vi "out_dc_unit.vi"(1 "input":T1) -> (0 "output":T2)   [LabVIEW 2013]
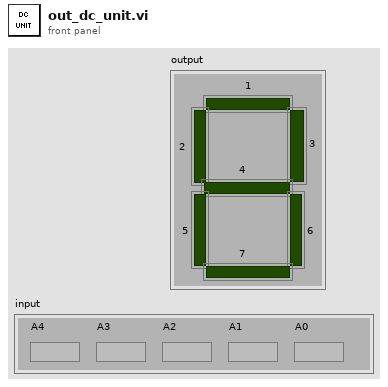
[diagram p1: front panel]
types:
  T1 = cluster{"A4":bool, "A3":bool, "A2":bool, "A1":bool, "A0":bool}
  T2 = cluster{"1":bool, "2":bool, "3":bool, "4":bool, "5":bool, "6":bool, "7":bool}
  T3 = cluster{bool, bool, bool, bool, bool, bool, bool}
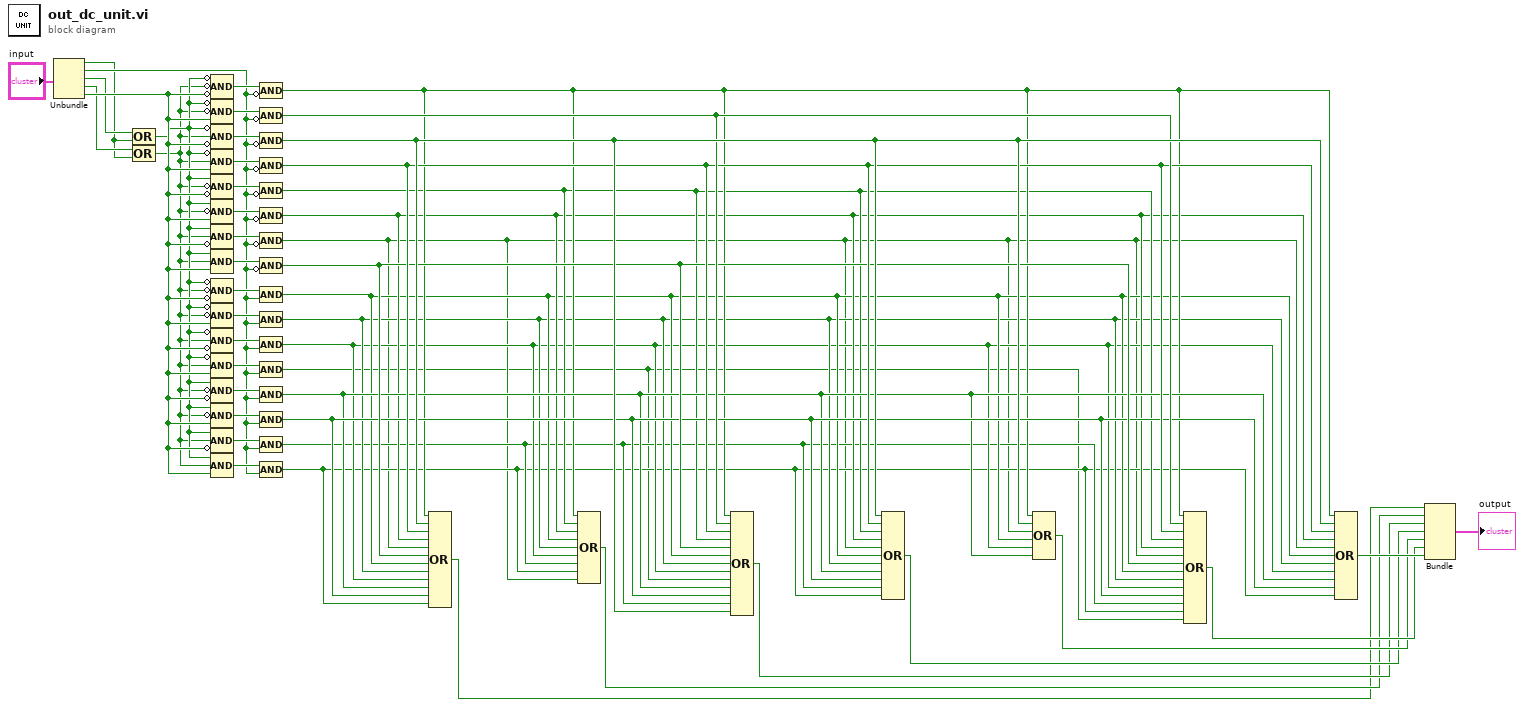
[diagram p0: block diagram]
diagram:
  n1 = Unbundle("input") -> ("A4"=w3:bool, "A3"=w6:bool, "A2"=w5:bool, "A1"=w4:bool, "A0"=w7:bool)
  n2 = Compound Arithmetic op=OR(w5, w3) -> (w2:bool)
  n3 = Compound Arithmetic op=OR(w4, w3) -> (w1:bool)
  n4 = Compound Arithmetic op=AND(invert w2, invert w1, invert w7) -> (w48:bool)
  n5 = Compound Arithmetic op=AND(invert w2, invert w1, w7) -> (w46:bool)
  n6 = Compound Arithmetic op=AND(invert w2, w1, invert w7) -> (w45:bool)
  n7 = Compound Arithmetic op=AND(invert w2, w1, w7) -> (w44:bool)
  n8 = Compound Arithmetic op=AND(w2, invert w1, invert w7) -> (w43:bool)
  n9 = Compound Arithmetic op=AND(w2, invert w1, w7) -> (w42:bool)
  n10 = Compound Arithmetic op=AND(w2, w1, invert w7) -> (w41:bool)
  n11 = Compound Arithmetic op=AND(w2, w1, w7) -> (w47:bool)
  n12 = Compound Arithmetic op=AND(invert w2, invert w1, invert w7) -> (w40:bool)
  n13 = Compound Arithmetic op=AND(invert w2, invert w1, w7) -> (w38:bool)
  n14 = Compound Arithmetic op=AND(invert w2, w1, invert w7) -> (w37:bool)
  n15 = Compound Arithmetic op=AND(invert w2, w1, w7) -> (w36:bool)
  n16 = Compound Arithmetic op=AND(w2, invert w1, invert w7) -> (w35:bool)
  n17 = Compound Arithmetic op=AND(w2, invert w1, w7) -> (w34:bool)
  n18 = Compound Arithmetic op=AND(w2, w1, invert w7) -> (w33:bool)
  n19 = Compound Arithmetic op=AND(w2, w1, w7) -> (w39:bool)
  n20 = Compound Arithmetic op=AND(w48, invert w6) -> (w19:bool)
  n21 = Compound Arithmetic op=AND(w46, invert w6) -> (w24:bool)
  n22 = Compound Arithmetic op=AND(w45, invert w6) -> (w25:bool)
  n23 = Compound Arithmetic op=AND(w44, invert w6) -> (w23:bool)
  n24 = Compound Arithmetic op=AND(w43, invert w6) -> (w18:bool)
  n25 = Compound Arithmetic op=AND(w42, invert w6) -> (w17:bool)
  n26 = Compound Arithmetic op=AND(w41, invert w6) -> (w11:bool)
  n27 = Compound Arithmetic op=AND(w47, invert w6) -> (w22:bool)
  n28 = Compound Arithmetic op=AND(w40, w6) -> (w16:bool)
  n29 = Compound Arithmetic op=AND(w38, w6) -> (w15:bool)
  n30 = Compound Arithmetic op=AND(w37, w6) -> (w14:bool)
  n31 = Compound Arithmetic op=AND(w36, w6) -> (w10:bool)
  n32 = Compound Arithmetic op=AND(w35, w6) -> (w20:bool)
  n33 = Compound Arithmetic op=AND(w34, w6) -> (w21:bool)
  n34 = Compound Arithmetic op=AND(w33, w6) -> (w13:bool)
  n35 = Compound Arithmetic op=AND(w39, w6) -> (w12:bool)
  n36 = Compound Arithmetic op=OR(w19, w25, w23, w17, w11, w22, w16, w15, w14, w20, w21, w12) -> (w26:bool)
  n37 = Compound Arithmetic op=OR(w19, w18, w17, w16, w15, w14, w13, w12, w11) -> (w27:bool)
  n38 = Compound Arithmetic op=OR(w19, w24, w23, w18, w22, w16, w15, w14, w10, w20, w21, w13, w25) -> (w28:bool)
  n39 = Compound Arithmetic op=OR(w25, w23, w18, w17, w11, w16, w15, w20, w21, w13, w12) -> (w29:bool)
  n40 = Compound Arithmetic op=OR(w19, w25, w11, w16, w14, w20) -> (w30:bool)
  n41 = Compound Arithmetic op=OR(w19, w24, w23, w18, w17, w11, w22, w16, w15, w14, w21, w13, w12, w10) -> (w31:bool)
  n42 = Compound Arithmetic op=OR(w19, w25, w23, w17, w11, w16, w15, w14, w20, w21, w12) -> (w32:bool)
  n43 = Bundle(w26, w27, w28, w29, w30, w31, w32) -> (→"output":T3)  [unwired: 1 in]
